vi "Help.vi"(8 "error in (no error)":errorcluster, 10 "Module name":string, 11 "Application Controller in":refnum<class "Application Controller.lvclass">) -> (0 "error out":errorcluster, 3 "Application Controller out":refnum<class "Application Controller.lvclass">)   [LabVIEW 2021, in "Application Controller.lvclass"]
uses:
  Application Controller.lvclass
  Application Controller.lvclass/Application Controller.ctl
  <vilib>/Platform/browser.llb/Open URL in Default Browser (path).vi
panel:
  out "Class name":string
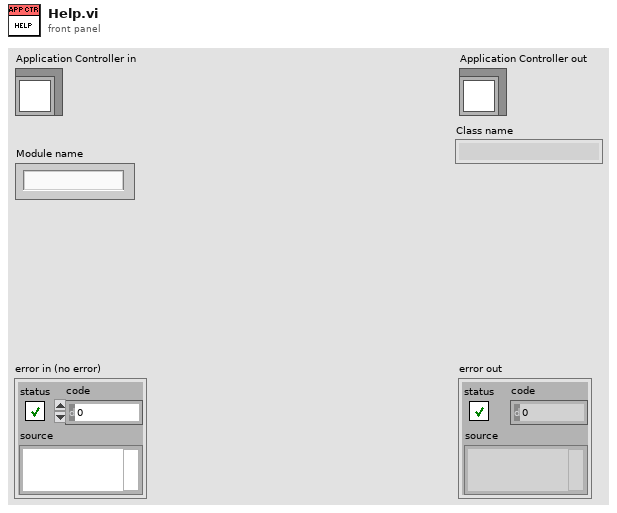
[diagram p1: front panel]
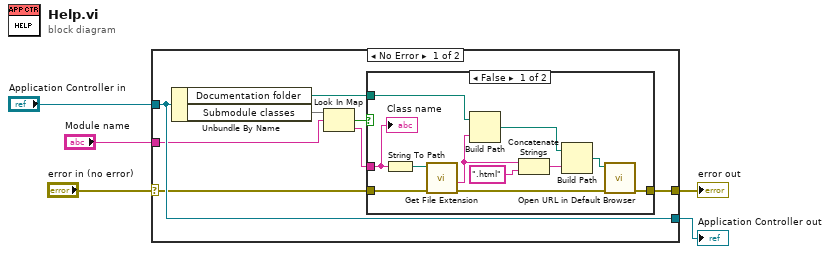
[diagram p0: block diagram]
diagram:
  n1 = case shown="No Error" "error in (no error)" {
    selector: "error in (no error)" -> [w7 w27]
    tunnel: [w6 w27] -> w4
    tunnel: [w13 w26] -> w2
    tunnel: "Application Controller in" -> [w13 w26]
    tunnel: "Module name" -> [w11 _]
    frame No Error {
      n2 = Unbundle By Name(w13) -> ("Documentation folder"=w8:path, "Submodule classes"=w12:map{string, string})
      n3 = Look In Map(map=w12, key=w11) -> (key not found?=w10:bool, value=w9:string)  [unwired: 1 in]
      n4 = case shown="False" w10 {
        tunnel: w9 -> [w24 _]
        tunnel: w8 -> [w22 _]
        tunnel: w7 -> [w16 w25]
        tunnel: [w14 w25] -> w6
        frame False {
          n5 = String To Path(string=w24) -> (path=w23:path)
          n6 = call <vilib>:"Get File Extension.vi"("error in (no error)"=w16, "file"=w23) -> ("error out"=w15:errorcluster, "filename without extension"=w21:string)  [unwired: 5 in, 3 out]
          n7 = Build Path(base path=w22, name or relative path=w21) -> (appended path=w19:path)
          n8 = Concatenate Strings(w21, ".html" ("string")) -> (w18:string)
          n9 = Build Path(base path=w19, name or relative path=w18) -> (appended path=w17:path)
          n10 = call-poly <vilib>:"Open URL in Default Browser.vi"("error in (no error)"=w15, "path"=w17) -> ("error out"=w14:errorcluster)  [unwired: 4 in, 1 out]
          "Class name" <- w24
        }
        frame True {
        }
      }
    }
    frame Error {
    }
  }
  "error out" <- w4
  "Application Controller out" <- w2
